vi "ParseCurrentPVResponce.vi"(11 "Responce":u8[](array[numeric])=[2, 48, 49, 82, 83, 68, 44, 79, 75, 44, 48, 48, 70, 65, 50, 51, 13, 10] format="%x") -> (2 "Current PV":dbl, 3 "Error Code":i8)   [LabVIEW 2015]
uses:
  <instrlib>/Samwontech TEMP2xxx/Samwontech TEMP2xxx.lvlib
panel:
  in  "Responce":string="\u000201RSD,OK,00FA23"
  out "Payload":string
  in  "Error Responce":u8[](array[numeric])=[2, 48, 49, 78, 71, 48, 49, 53, 55, 13, 10] format="%x"
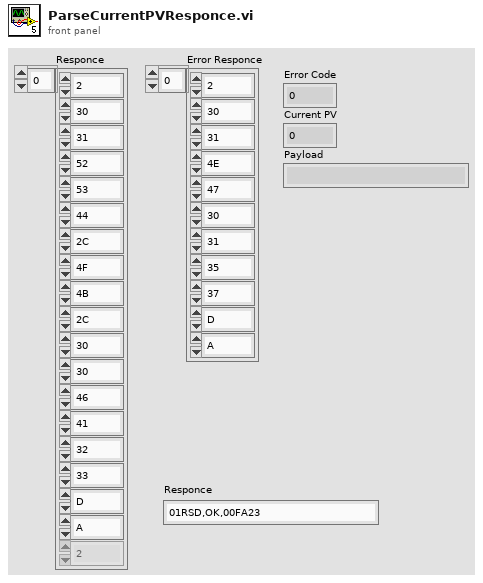
[diagram p1: front panel]
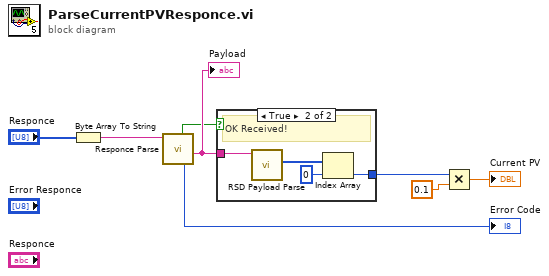
[diagram p0: block diagram]
diagram:
  n1 = Byte Array To String(unsigned byte array="Responce") -> (string=w8:string)
  n2 = call <instrlib>:"Responce Parse.vi"("Responce"=w8) -> ("Payload"=w7:string, "Error Code"=→"Error Code":i8, "OK"=w6:bool)  [unwired: 4 in, 4 out]
  "Payload" <- w7
  n3 = case shown="True" w6 {
    tunnel: [_ w9] -> w3
    tunnel: w7 -> [_ w10]
    frame False {
    }
    frame True {
      # "OK Received!"
      n4 = call <instrlib>:"RSD Payload Parse.vi"("Payload"=w10) -> ("Data (number)"=w12:i16[])  [unwired: 9 in, 1 out]
      n5 = Index Array(array=w12, index=0) -> (element=w9:i16)
    }
  }
  n6 = Multiply(x=w3, y=0.1) -> (x*y=→"Current PV":dbl)
